vi "Read Device Information.vi"(6 "timeout ms (1000)":i32=1000, 8 "error in (no error)":errorcluster, 10 "Conformity Level":enum8{"None", "Basic", "Regular", "Extended"}(ring)=enum."Regular", 11 "TCP Network Connection in":refnum<k5>) -> (0 "error in (no error) 2":errorcluster, 2 "Objects":T1(array[cluster]), 3 "TCP Network Connection out":refnum<k5>)   [LabVIEW 2023, in "Modbus TCP Micro.lvlib"]
uses:
  Modbus TCP Micro.lvlib
  Modbus Functions.ctl
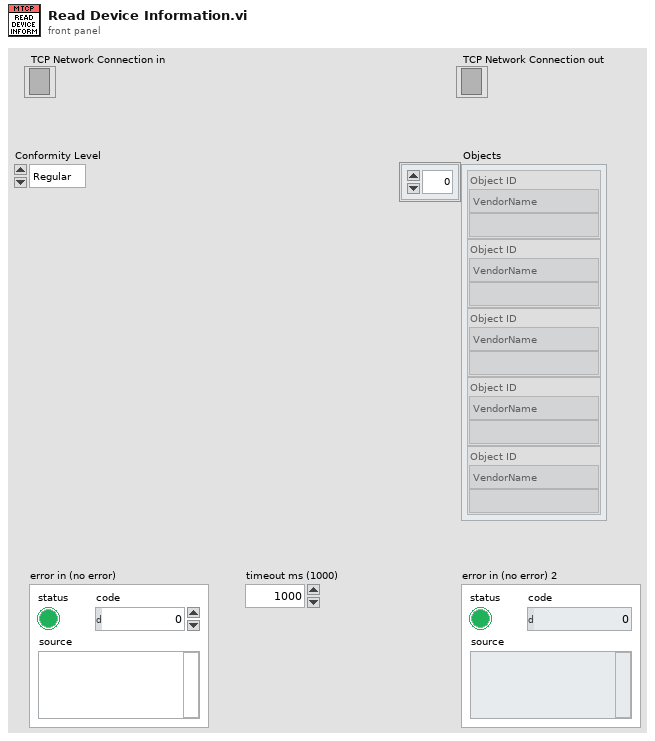
[diagram p1: front panel]
types:
  T1 = cluster{"Object ID":enum8{"VendorName", "ProductCode", "MajorMinorRevision", "VendorUrl", "ProductName", "ModelName", "UserApplicationName"}, "String":string}[]
  T2 = cluster{"ReadDevID Code":u8, "Conformity Level":u8, "MoreFollows":u8, "Next Object ID":u8, "Number of Objects":u8}
  T3 = typedef "Modbus TCP Micro.lvlib/Modbus Functions.ctl" = u8
  T4 = cluster{"Object ID":enum8{"VendorName", "ProductCode", "MajorMinorRevision", "VendorUrl", "ProductName", "ModelName", "UserApplicationName"}, "Object Length":u8}
  T5 = enum8{"VendorName", "ProductCode", "MajorMinorRevision", "VendorUrl", "ProductName", "ModelName", "UserApplicationName"}
  T6 = cluster{"Object ID":enum8{"VendorName", "ProductCode", "MajorMinorRevision", "VendorUrl", "ProductName", "ModelName", "UserApplicationName"}, string}
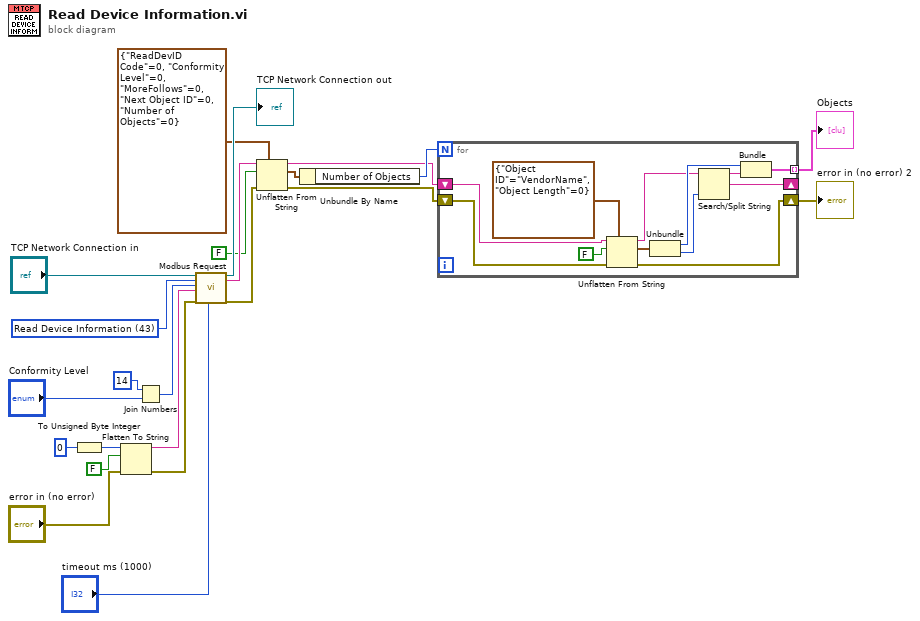
[diagram p0: block diagram]
diagram:
  w21 = T3 43 items=["None"=0, "Read Coil Status"=1, "Read Input Status"=2, "Read Holding Registers"=3, "Read Input Registers"=4, "Force Single Coil"=5, "Preset Single Register"=6, "Force Multiple Coils"=15, "Preset Multiple Registers"=16, "Mask Write Register"=22, "Read Write Registers"=23, "Read Device Information"=43] ("Function Codes")
  n1 = To Unsigned Byte Integer(number=u8 0) -> (unsigned 8bit integer=w14:u8)
  n2 = Flatten To String(anything=w14, prepend array or string size? (T)=FALSE, error in (no error)="error in (no error)") -> (data string=w13:string, error out=w15:errorcluster)  [unwired: 1 in, 1 out]
  n3 = Join Numbers(hi=u8 14, lo="Conformity Level") -> ((hi.lo)=w16:u16)
  n4 = call "Modbus Request.vi"("TCP Network Connection in"="TCP Network Connection in", "Function Codes"=w21, "Start Address"=w16, "Payload"=w13, "error in (no error)"=w15, "timeout ms (1000)"="timeout ms (1000)") -> ("TCP Network Connection out"=→"TCP Network Connection out":refnum<k5>, "Payload"=w9:string, "error out"=w19:errorcluster)  [unwired: 8 in, 3 out]
  n5 = Unflatten From String(type=T2 {"ReadDevID Code"=0, "Conformity Level"=0, "MoreFollows"=0, "Next Object ID"=0, "Number of Objects"=0}, binary string=w9, data includes array or string size? (T)=FALSE, error in (no error)=w19) -> (rest of the binary string=w4:string, value=w1:T2, error out=w10:errorcluster)  [unwired: 1 in]
  n6 = Unbundle By Name(w1) -> ("Number of Objects"=w6:u8)
  n7 = for {
    N: w6 -> [_]
    shift-right: [w34] -> w7
    shift-left: w10 -> [w35]
    shift-right: [w24] -> _
    shift-left: w4 -> [w32]
    tunnel: [w29] -> w3 mode=indexing
    n8 = Unflatten From String(type=T4 {"Object ID"=enum."VendorName", "Object Length"=0}, binary string=w32, data includes array or string size? (T)=FALSE, error in (no error)=w35) -> (rest of the binary string=w27:string, value=w28:T4, error out=w34:errorcluster)  [unwired: 1 in]
    n9 = Unbundle(w28) -> ("Object ID"=w30:T5, "Object Length"=w26:u8)
    n10 = Search/Split String(string=w27, offset (0)=w26) -> (substring before match=w25:string, match + rest of string=w24:string)  [unwired: 1 in, 1 out]
    n11 = Bundle("Object ID"=w30, w25) -> (w29:T6)  [unwired: 1 in]
  }
  "error in (no error) 2" <- w7
  "Objects" <- w3
